vi "Object_Track_Webcam_RIO.vi"() -> ()   [LabVIEW 2017]
doc: "This example demonstrates the Traditional MeanShift algorithm to track an object in the image."
uses:
  <vilib>/userdefined/High Color/IMAQdx.ctl
  <vilib>/vision/driver/NI_Vision_Acquisition_Software.lvlib
panel:
  out "CPU Load":dbl(graph)
  in  "Camera Select":T1="cam0"
  out "Distance":dbl
  in  "Stop":bool
  out "Image":T2(plugin-control)
  # "Overview: Demonstrate the Traditional MeanShift algorithm to track an object in the image.\nRequirements: LabVIEW Full Development System and Vision Development Module.\nInstructions: Run the VI."
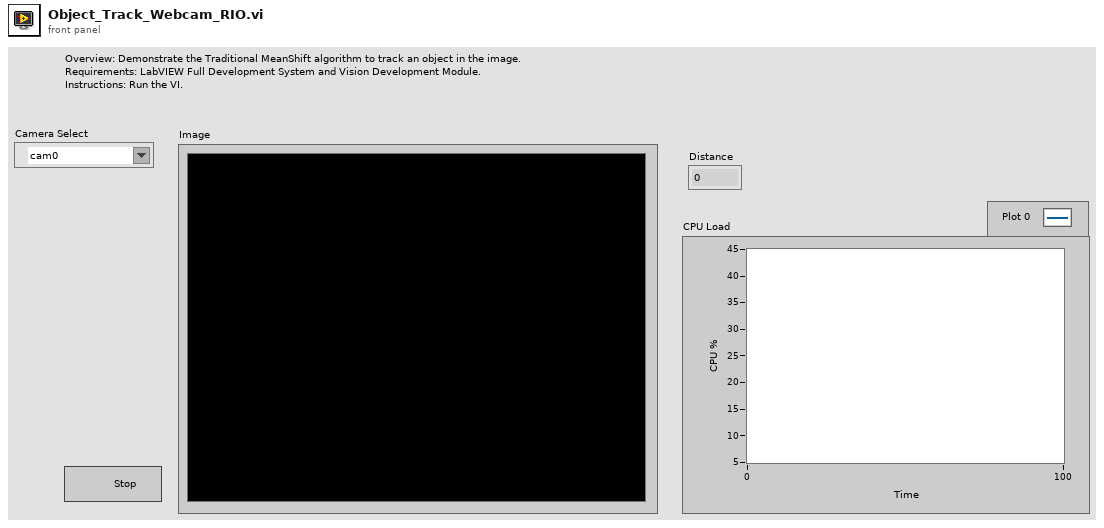
[diagram p1: front panel]
types:
  T1 = typedef "IMAQdx.ctl" = refnum<k21>
  T2 = typedef "IMAQ Image.ctl" = refnum<image>
  T3 = typedef "Image Type" = u32
  T4 = cluster{"Number of Histogram Bins":i32, "Blending Parameter (%)":dbl, "Maximum Iterations":i32}
  T5 = typedef "IMAQ Object Tracking Session.ctl" = refnum<k20>
  T6 = typedef "IMAQ Point" = cluster{"X":sgl, "Y":sgl}
  T7 = typedef "ROI Descriptor" = cluster{"Global Rectangle":i32[], "Contours":cluster{"ID":enum32{"External", "Internal"}, "Type":u32, "Coordinates":i32[]}[]}
  T8 = cluster{"Label":string, "Score":i32, "Angle":dbl, "Location":cluster{"X":dbl, "Y":dbl}, "Bounding Box":cluster{"X":dbl, "Y":dbl}[], "Object Found?":bool}[]
  T9 = cluster{"Label":string, "Score":i32, "Angle":dbl, "Location":cluster{"X":dbl, "Y":dbl}, "Bounding Box":cluster{"X":dbl, "Y":dbl}[], "Object Found?":bool}
  T10 = cluster{"Desired Font (Application)":enum16{"User-specified Font", "Application Font", "System Font", "Dialog Font"}, "[User-specified Font]":cluster{"Font Name":string, "Size":i16, "Strikeout?":bool, "Italic?":bool, "Underline?":bool, "Outline?":bool, "Shadow?":bool, "Bold?":bool, "Rotation Angle":dbl}, "Horizontal Alignment":i16, "Vertical Alignment":i16}
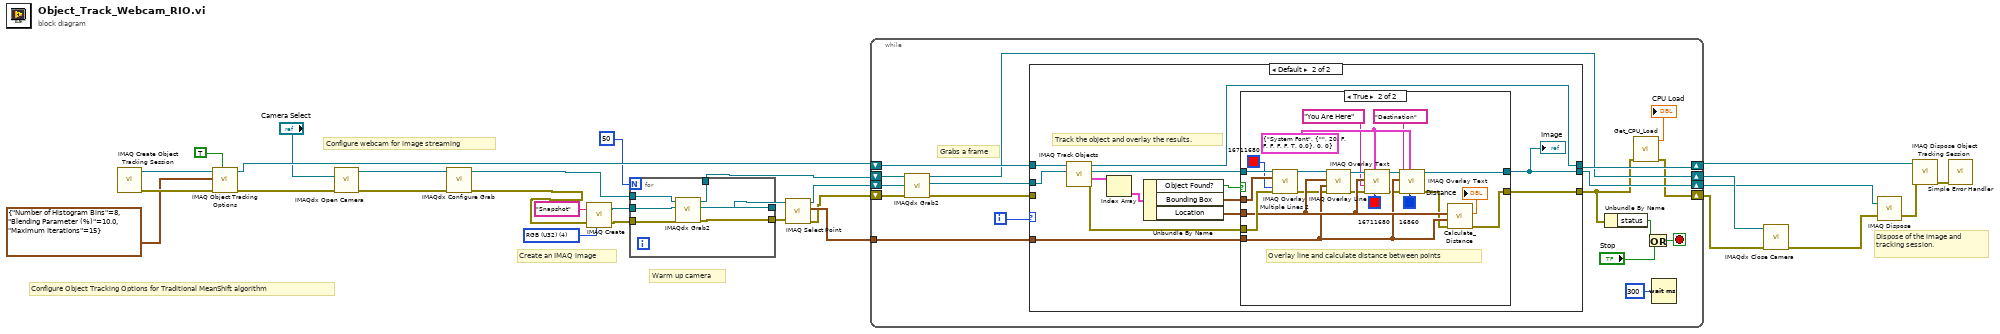
[diagram p0: block diagram]
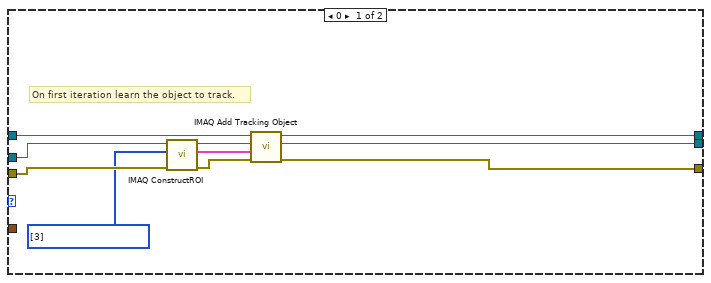
[diagram p2: hidden frame]
diagram:
  w21 = T3 4 items=["Grayscale (U8)", "Grayscale (I16)", "Grayscale (SGL)", "Complex (CSG)", "RGB (U32)", "HSL (U32)", "RGB (U64)", "Grayscale (U16)"] ("Image Type")
  # "Warm up camera"
  # "Create an IMAQ image"
  # "Configure webcam for image streaming"
  # "Configure Object Tracking Options for Traditional MeanShift algorithm"
  # "Dispose of the image and tracking session."
  n1 = call "IMAQ Create Object Tracking Session"() -> ("error out"=w24:errorcluster, "Object Tracking Session"=w26:T5)  [unwired: 1 in, 9 out]
  n2 = call-poly "IMAQ Object Tracking Options"("Get/Set (Get)"=TRUE, "error in (no error)"=w24, "Mean Shift Options in"=T4 {"Number of Histogram Bins"=8, "Blending Parameter (%)"=10.0, "Maximum Iterations"=15}, "Object Tracking Session In"=w26) -> ("error out"=w20:errorcluster, "Object Tracking Session Out"=w17:T5)  [unwired: 5 in, 1 out]
  n3 = call <vilib>:"IMAQdx Open Camera.vi"("error in"=w20, "Session In"="Camera Select") -> ("error out"=w19:errorcluster, "Session Out"=w6:T1)  [unwired: 8 in]
  n4 = call <vilib>:"IMAQdx Configure Grab.vi"("error in"=w19, "Session In"=w6) -> ("error out"=w2:errorcluster, "Session Out"=w1:T1)  [unwired: 8 in]
  n5 = call "IMAQ Create"("Image Name"="Snapshot", "Image Type"=w21, "error in (no error)"=w2) -> ("New Image"=w14:T2, "error out"=w13:errorcluster)  [unwired: 2 in]
  n6 = for {
    N: 50 -> [_]
    tunnel: w1 -> [w35]
    tunnel: w14 -> [w34]
    tunnel: w13 -> [w33]
    tunnel: [w32] -> w11
    tunnel: [w31] -> w10
    tunnel: [w30] -> w4
    n7 = call <vilib>:"IMAQdx Grab2.vi"("error in"=w33, "Image In"=w34, "Session In"=w35) -> ("error out"=w32:errorcluster, "Image Out"=w31:T2, "Session Out"=w30:T1)  [unwired: 5 in, 1 out]
  }
  n8 = call "IMAQ Select Point"("error in (no error)"=w11, "Image In"=w10) -> ("error out"=w3:errorcluster, "Point"=w9:T6, "Image Out (duplicate)"=w8:T2)  [unwired: 6 in, 1 out]
  n9 = while {
    shift-right: [w50] -> w29
    shift-left: w17 -> [w51]
    shift-right: [w38] -> w15
    shift-left: w3 -> [w47]
    shift-right: [w43] -> w16
    shift-left: w4 -> [w46]
    tunnel: w9 -> [w40]
    shift-right: [w52] -> w12
    shift-left: w8 -> [w41]
    i -> [w45]
    stop <- w48 stop-if-true
    # "Grabs a frame"
    n10 = call <vilib>:"IMAQdx Grab2.vi"("error in"=w47, "Image In"=w41, "Session In"=w46) -> ("error out"=w44:errorcluster, "Image Out"=w37:T2, "Session Out"=w43:T1)  [unwired: 5 in, 1 out]
    n11 = case shown="Default" w45 {
      tunnel: [w60 w76] -> w50
      tunnel: [w62 w67] -> w52
      tunnel: [w61 w68] -> w39
      tunnel: w51 -> [w63 w72]
      tunnel: w37 -> [w54 w69]
      tunnel: w44 -> [w57 _]
      tunnel: w40 -> [_ w65]
      frame 0 {
        w55 = u32[] [3] items=["No Selection", "Point", "Line", "Rectangle", "Oval", "Polygon", "Freehand Region", "Annulus", "Zoom", "Pan", "Broken Line", "Freehand Line", "Rotated Rectangle"] ("Tools")
        # "On first iteration learn the object to track."
        n12 = call "IMAQ ConstructROI"("error in (no error)"=w57, "Tools"=w55, "Image"=w54) -> ("error out"=w56:errorcluster, "ROI Descriptor Out"=w58:T7, "Image Out (duplicate)"=w59:T2)  [unwired: 5 in, 1 out]
        n13 = call "IMAQ Add Tracking Object"("error in (no error)"=w56, "ROI Descriptor"=w58, "Image"=w59, "Object Tracking Session In"=w63) -> ("error out"=w61:errorcluster, "Image (duplicate)"=w62:T2, "Object Tracking Session Out"=w60:T5)  [unwired: 1 in, 4 out]
      }
      frame Default {
        # "Track the object and overlay the results."
        n14 = call "IMAQ Track Objects"("Image"=w69, "Object Tracking Session In"=w72) -> ("error out"=w71:errorcluster, "Objects (pixel)"=w75:T8, "Image (duplicate)"=w74:T2, "Object Tracking Session Out"=w76:T5)  [unwired: 2 in, 4 out]
        n15 = Index Array(array=w75) -> (element=w70:T9)  [unwired: 1 in]
        n16 = Unbundle By Name(w70) -> ("Object Found?"=w64:bool, "Bounding Box"=w73:cluster{"X":dbl, "Y":dbl}[], "Location"=w66:cluster{"X":dbl, "Y":dbl})
        n17 = case shown="True" w64 {
          tunnel: w74 -> [w78 w99]
          tunnel: w73 -> [_ w98]
          tunnel: w71 -> [w77 w97]
          tunnel: [w77 w96] -> w68
          tunnel: [w78 w95] -> w67
          tunnel: w66 -> [_ w94]
          tunnel: w65 -> [_ w93]
          frame False {
          }
          frame True {
            w82 = T10 {"Desired Font (Application)"=enum."System Font", "[User-specified Font]"={"Font Name"="", "Size"=20, "Strikeout?"=FALSE, "Italic?"=FALSE, "Underline?"=FALSE, "Outline?"=FALSE, "Shadow?"=FALSE, "Bold?"=TRUE, "Rotation Angle"=0.0}, "Horizontal Alignment"=0, "Vertical Alignment"=0} ("Font, Size & Style")
            # "Overlay line and calculate distance between points"
            n18 = call "IMAQ Overlay Multiple Lines 2"("Image"=w99, "Line End Points"=w98, "Color"=u32 16711680, "error in (no error)"=w97) -> ("Image Out"=w90:T2, "error out"=w89:errorcluster)  [unwired: 4 in, 6 out]
            n19 = call "IMAQ Overlay Line"("error in (no error)"=w89, "End Point"=w93, "Start Point"=w94, "Image"=w90) -> ("error out"=w83:errorcluster, "Image Out"=w84:T2)  [unwired: 6 in]
            n20 = call "IMAQ Overlay Text"("Text Color (black)"=u32 16711680, "Font, Size & Style"=w82, "error in (no error)"=w83, "String"="You Are Here", "Origin"=w94, "Image"=w84) -> ("error out"=w86:errorcluster, "Image Out"=w85:T2)  [unwired: 4 in]
            n21 = call "IMAQ Overlay Text"("Text Color (black)"=u32 16860, "Font, Size & Style"=w82, "error in (no error)"=w86, "String"="Destination", "Origin"=w93, "Image"=w85) -> ("error out"=w80:errorcluster, "Image Out"=w95:T2)  [unwired: 4 in]
            n22 = call "Calculate_Distance.vi"("error in (no error)"=w80, "Destination"=w93, "Position"=w94) -> ("error out"=w96:errorcluster, "Distance"=→"Distance":dbl)  [unwired: 7 in]
          }
        }
        "Image" <- w67
      }
    }
    n23 = Unbundle By Name(w39) -> ("status"=w53:bool)
    n24 = call "Get_CPU_Load.vi"("error in (no error)"=w39) -> ("error out"=w38:errorcluster, "Numeric"=→"CPU Load":dbl)  [unwired: 9 in]
    n25 = Or(x=w53, y="Stop") -> (x .or. y?=w48:bool)
    n26 = Wait (ms)(milliseconds to wait=u32 300) -> ()  [unwired: 1 out]
  }
  n27 = call <vilib>:"IMAQdx Close Camera.vi"("error in"=w15, "Session In"=w16) -> ("error out"=w18:errorcluster)  [unwired: 9 in]
  n28 = call "IMAQ Dispose"("Image"=w12, "error in (no error)"=w18) -> ("error out"=w28:errorcluster)  [unwired: 1 in, 3 out]
  n29 = call "IMAQ Dispose Object Tracking Session"("error in (no error)"=w28, "Object Tracking Session"=w29) -> ("error out"=w27:errorcluster)  [unwired: 9 out]
  n30 = call <vilib>:"Simple Error Handler.vi"("error in (no error)"=w27) -> ()  [unwired: 1 in, 8 out]
